vi "GV preline gate.vi"() -> ()   [LabVIEW 2017]
panel:
  out "Preline Gate":bool
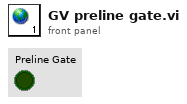
[diagram p1: front panel]
diagram:
